vi "Set Multi Track.vi"(6 "gap":i32, 7 "bottom":i32, 8 "error in (no error)":errorcluster, 9 "offset":i32, 10 "height":i32, 11 "number":i32) -> (0 "error out":errorcluster, 3 "function return":u32, 4 "gap out":i32, 5 "bottom out":i32)   [LabVIEW 2014, in "atmcd32d.lvlib"]
doc: "unsigned int WINAPI SetMultiTrack(int number, int height, int offset, int * bottom, int * gap);"
uses:
  atmcd32d.lvlib
  atmcd32d.dll
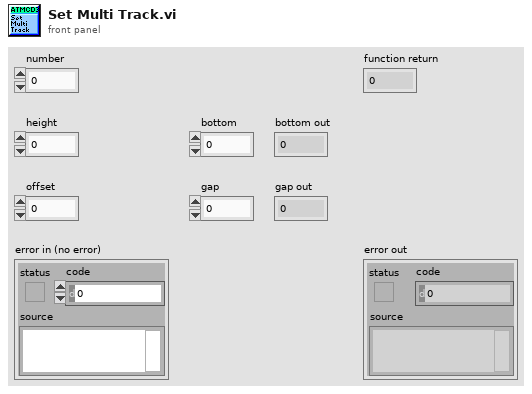
[diagram p1: front panel]
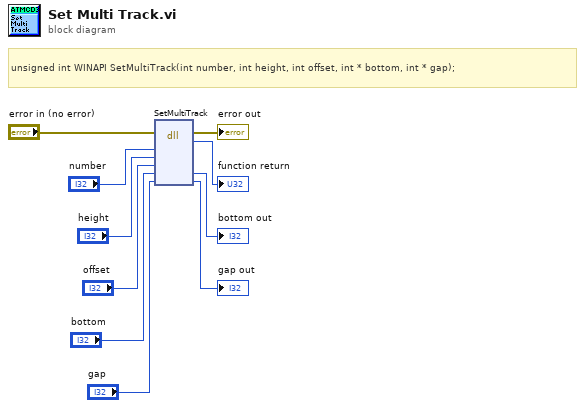
[diagram p0: block diagram]
diagram:
  # "unsigned int WINAPI SetMultiTrack(int number, int height, int offset, int * bottom, int * gap);"
  n1 = dll-call lib="C:/Users/Bakir/Documents/Lambda2-Testing/lib/Andorlib/atmcd32d.*" fn="SetMultiTrack"(error in="error in (no error)", "number"="number", "height"="height", "offset"="offset", "bottom"="bottom", "gap"="gap") -> (error out=→"error out":errorcluster, →"function return":u32, "bottom"=→"bottom out":i32, "gap"=→"gap out":i32)  [unwired: 5 in, 1 out]
